vi "array dimension array - array 1D template.vi"() -> ()   [LabVIEW 2012]
panel:
  out "Array Size":i32[](array[numeric])
  in  "Array":dbl[](array[numeric])
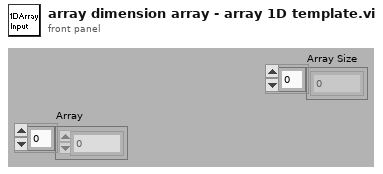
[diagram p1: front panel]
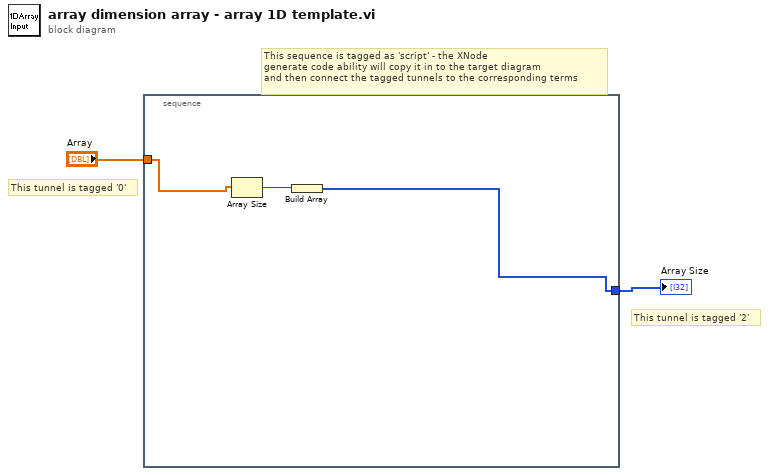
[diagram p0: block diagram]
diagram:
  # "This tunnel is tagged '2'"
  # "This tunnel is tagged '0'"
  # "This sequence is tagged as 'script' - the XNode \ngenerate code ability will copy it in to the target diagram\nand then connect the tagged tunnels to the corresponding terms"
  n1 = stacked-sequence {
    tunnel: "Array" -> [w5]
    tunnel: [w3] -> w1
    frame #0 {
      n2 = Array Size(array=w5) -> (size(s)=w4:i32)
      n3 = Build Array(w4) -> (w3:i32[])
    }
  }
  "Array Size" <- w1
